vi "ConfigTCS.vi"() -> ()   [LabVIEW 2011]
uses:
  <vilib>/Utility/config.llb/Read Key (String).vi
  <vilib>/Utility/config.llb/Read Key (U32).vi
  SerialCommError.vi
  <vilib>/Instr/_visa.llb/VISA Configure Serial Port (Instr).vi
  <vilib>/Utility/config.llb/NI_LVConfig.lvlib
panel:
  out "Connected?":bool
  out "CommType":string
  out "properties.ini":path=path "C:/BonOMM/BonOMM 7.1/BonOMM 7.1.vi" caption="Fichier de Configuration Système"
  out "VISA resource name":refnum<visa-resource-name>
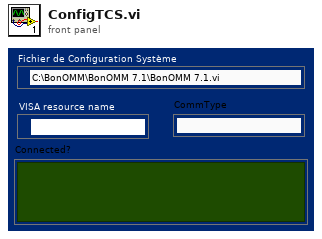
[diagram p1: front panel]
types:
  T1 = typedef "NI_LVConfig.lvlib/Config Data RefNum.ctl" = refnum<k1>
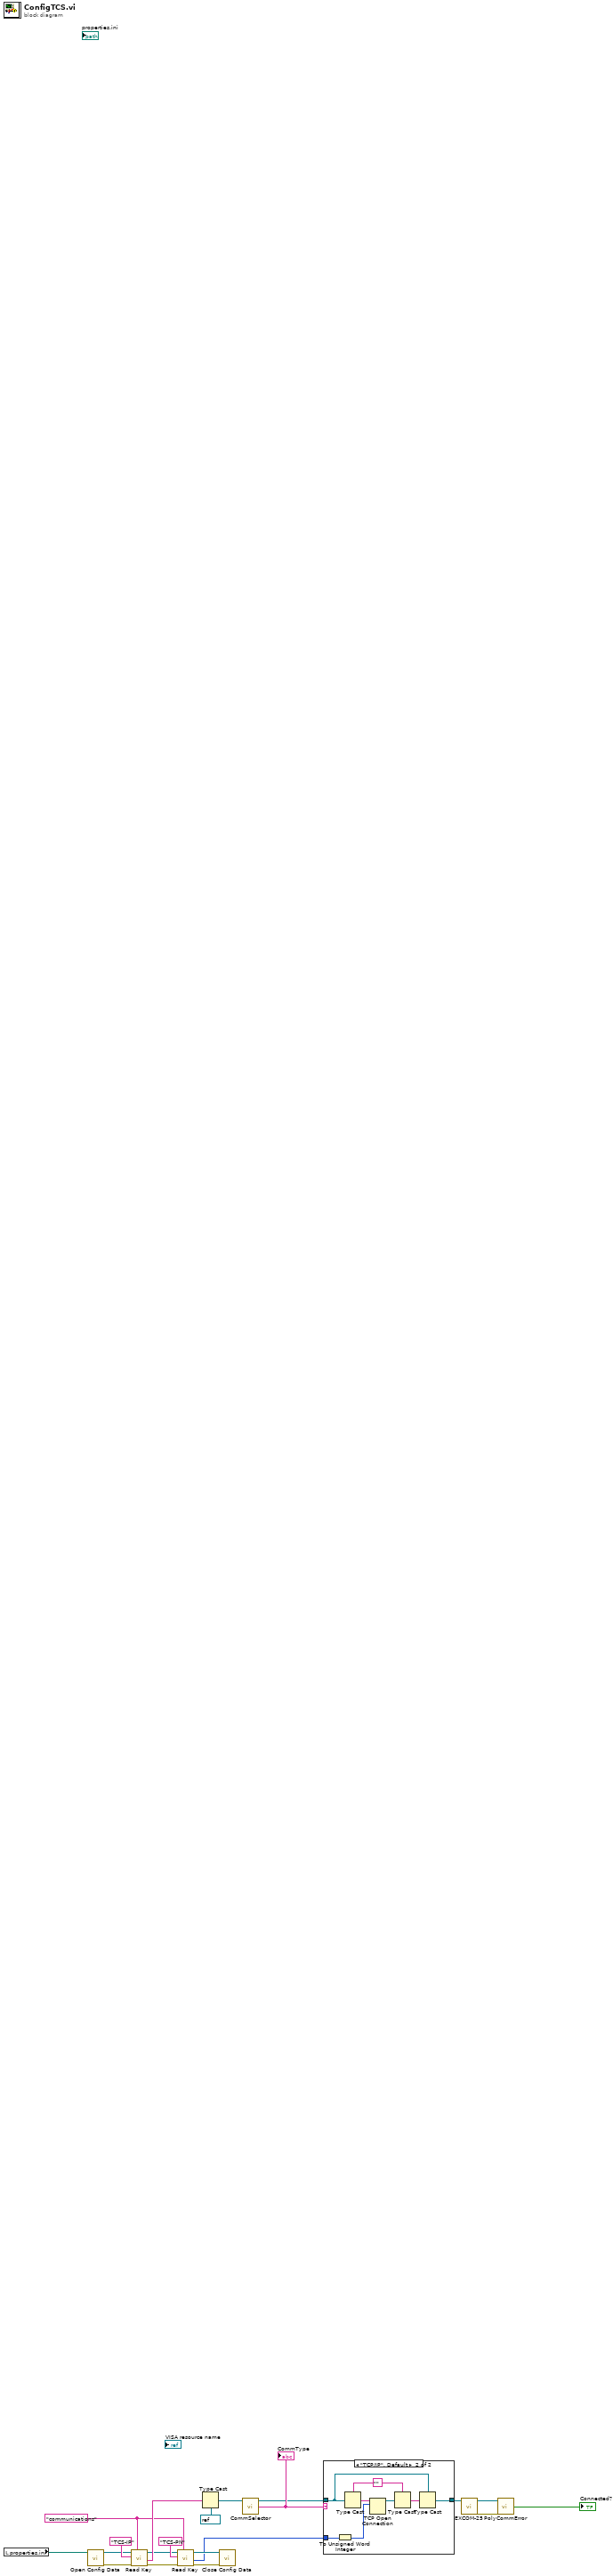
[diagram p0: block diagram]
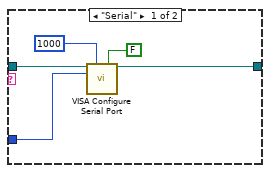
[diagram p2: hidden frame]
diagram:
  w16 = "communications" ("name or relative path")
  n1 = local read "properties.ini"() -> (w8:path)
  n2 = call <vilib>:"Open Config Data.vi"("configuration file path"=w8) -> ("error out"=w11:errorcluster, "refnum"=w10:T1)  [unwired: 8 in, 1 out]
  n3 = call-poly <vilib>:"Read Key.vi"("section"=w16, "error in (no error)"=w11, "key"="TCS-IP" ("name or relative path"), "refnum"=w10) -> ("error out"=w13:errorcluster, "value"=w19:string, "refnum out"=w12:T1)  [unwired: 4 in, 1 out]
  n4 = call-poly <vilib>:"Read Key.vi"("section"=w16, "error in (no error)"=w13, "key"="TCS-PN" ("name or relative path"), "refnum"=w12) -> ("error out"=w15:errorcluster, "value"=w5:u32, "refnum out"=w14:T1)  [unwired: 4 in, 1 out]
  n5 = Type Cast(type=refnum<visa-resource-name> "-1" ("TCS R VRN"), x=w19) -> (*(type *) &x=w9:refnum<visa-resource-name>)
  n6 = call <vilib>:"Close Config Data.vi"("error in (no error)"=w15, "refnum"=w14) -> ()  [unwired: 8 in, 2 out]
  n7 = call "CommSelector.vi"("VISA resource name"=w9) -> ("VISA resource name"=w6:refnum<visa-resource-name>, "CommType"=w7:string)  [unwired: 13 in]
  "CommType" <- w7
  n8 = case shown="\"TCP/IP\", Default" w7 {
    tunnel: w6 -> [w23 w28]
    tunnel: w5 -> [w22 w27]
    tunnel: [w21 w29] -> w4
    frame "Serial" {
      n9 = call-poly "VISA Configure Serial Port"("VISA resource name"=w23, "timeout (10sec)"=u32 1000, "Enable Termination\nChar (T)"=FALSE ("Enable Termination\nChar (T)"), "baud rate (9600)"=w22) -> ("VISA resource name out"=w21:refnum<visa-resource-name>)  [unwired: 10 in, 1 out]
    }
    frame "TCP/IP", Default {
      w31 = ""
      n10 = To Unsigned Word Integer(number=w27) -> (unsigned 16bit integer=w26:u16)
      n11 = Type Cast(type=w31, x=w28) -> (*(type *) &x=w33:string)
      n12 = TCP Open Connection(address=w33, remote port or service name=w26) -> (connection ID=w32:refnum<k5>)  [unwired: 3 in, 1 out]
      n13 = Type Cast(type=w31, x=w32) -> (*(type *) &x=w30:string)
      n14 = Type Cast(type=w28, x=w30) -> (*(type *) &x=w29:refnum<visa-resource-name>)
    }
  }
  n15 = call "EXCOM-25.vi"("VISA resource name"=w4) -> ("VISA resource name dup"=w3:refnum<visa-resource-name>, "Error OUT"=w2:errorcluster)  [unwired: 4 in, 13 out]
  n16 = call-poly "PolyCommError.vi"("VISA IN"=w3, "error IN"=w2) -> ("Boolean"=→"Connected?":bool)  [unwired: 11 in, 2 out]
